vi "Add.vi"(1 "x":sgl, 2 "y":sgl, 4 "Adder4":refnum<class "Adder4.lvclass">) -> (6 "x+y":sgl)   [LabVIEW 2017, in "Adder4.lvclass"]
uses:
  Adder4.lvclass
  Adder.lvclass
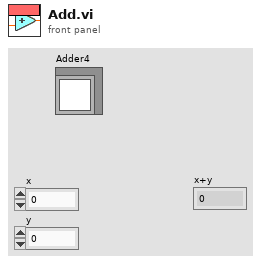
[diagram p1: front panel]
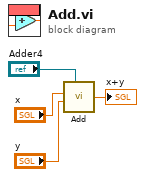
[diagram p0: block diagram]
diagram:
  n1 = call-parent "Add.vi"("x"="x", "y"="y", "Adder"="Adder4") -> ("x+y"=→"x+y":sgl)  [unwired: 4 in]
